vi "Get_Input_Trigger_Mode.vi"(8 "error in (no error)":errorcluster, 11 ".NET Reference in":refnum<k24>) -> (0 "error out":errorcluster, 2 "mode":enum16{"Disable", "Enable", ""}(ring), 3 ".NET Reference out":refnum<k24>)   [LabVIEW 2017]
uses:
  LV_IL_Sample/DLL/InstrumentDLL.dll
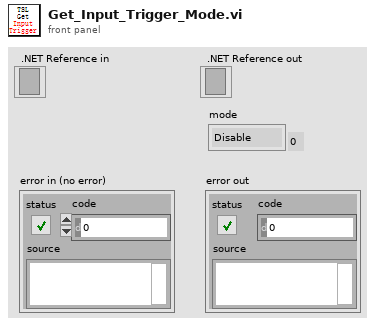
[diagram p1: front panel]
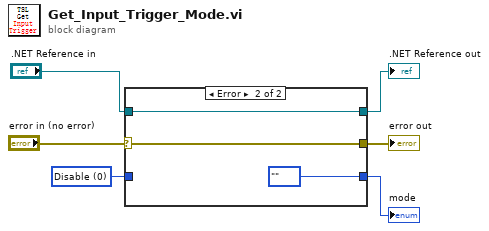
[diagram p0: block diagram]
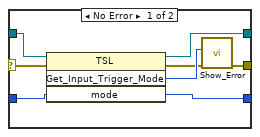
[diagram p2: hidden frame]
diagram:
  w3 = 0 items=["Disable", "Enable"] ("mode")
  n1 = case shown="Error" "error in (no error)" {
    selector: "error in (no error)" -> [w8 w17]
    tunnel: [w9 w17] -> w6
    tunnel: [w14 w16] -> w5
    tunnel: ".NET Reference in" -> [w13 w16]
    tunnel: w3 -> [w12 _]
    tunnel: [w7 enum16{"Disable", "Enable", ""}."" ("mode")] -> w1
    frame No Error {
      n2 = invoke on="调用节点" class="TSL" method="Get_Input_Trigger_Mode"(reference=w13, error in=w8, "mode"=w12) -> (reference out=w14:refnum<k24>, error out=w10:errorcluster, "Get_Input_Trigger_Mode"=w11:i32, "mode"=w7:i32)  [unwired: 1 in]
      n3 = call "Show_Error.vi"("error in (no error)"=w10, "Error"=w11) -> ("error out"=w9:errorcluster)  [unwired: 9 in]
    }
    frame Error {
    }
  }
  "error out" <- w6
  ".NET Reference out" <- w5
  "mode" <- w1
